vi "GetDocument.vi"(0 "reference in":refnum<class "LcWebView.lvclass">, 5 "Error In":errorcluster) -> (14 "reference out":refnum<class "LcWebView.lvclass">, 15 "Result":string, 19 "Error Out":errorcluster)   [LabVIEW 2021, in "LcWebView.lvclass"]
doc: "Get HTML comtent"
uses:
  LcWebView.lvclass
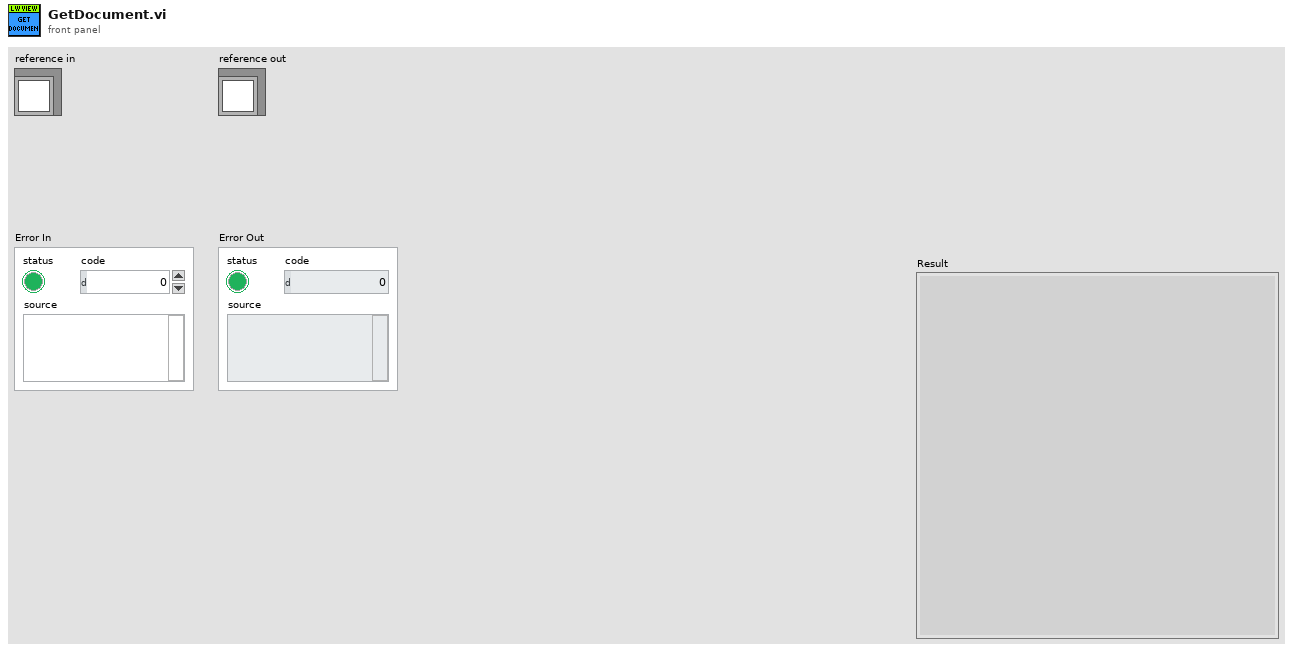
[diagram p1: front panel]
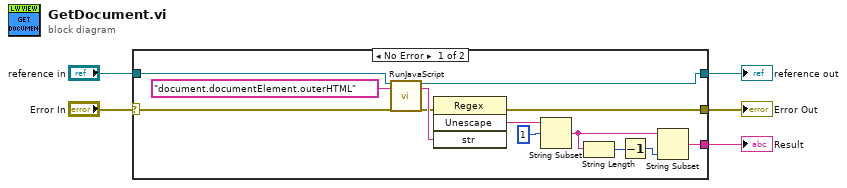
[diagram p0: block diagram]
diagram:
  n1 = case shown="No Error" "Error In" {
    selector: "Error In" -> [w16 w20]
    tunnel: [w6 w20] -> w4
    tunnel: [w15 w19] -> w2
    tunnel: "reference in" -> [w18 w19]
    tunnel: [w8 _] -> w1
    frame No Error {
      n2 = call-dynamic "RunJavaScript.vi"("reference in"=w18, "Java Script Function"="document.documentElement.outerHTML" ("javaScript"), "Error In"=w16) -> ("reference out"=w15:refnum<class "LcWebView.lvclass">, "Result"=w14:string, "Error Out"=w7:errorcluster)  [unwired: 13 in, 1 out]
      n3 = invoke class="Regex" method="Unescape"(error in=w7, "str"=w14) -> (error out=w6:errorcluster, "Unescape"=w9:string)  [unwired: 2 in, 2 out]
      n4 = String Subset(string=w9, offset (0)=1) -> (substring=w12:string)  [unwired: 1 in]
      n5 = String Length(string=w12) -> (length=w11:i32)
      n6 = Decrement(x=w11) -> (x-1=w10:i32)
      n7 = String Subset(string=w12, length (rest)=w10) -> (substring=w8:string)  [unwired: 1 in]
    }
    frame Error {
    }
  }
  "Error Out" <- w4
  "reference out" <- w2
  "Result" <- w1
